vi "35Cl + 37Cl inj - 35Cl HE.vi"(6 "measure transmission?":bool, 7 "na/V 2":dbl=5000.0, 8 "error in":errorcluster, 9 "measure ss":bool=TRUE, 10 "field change wait(s)":u32=8, 11 "na/V":dbl=1000.0) -> (0 "error out":errorcluster, 1 "stable current 2":dbl format="%.2f", 3 "stable current":dbl=0.03723971270335772 format="%.2f", 4 "inj current":dbl format="%#_6e", 5 "INJ ss ratio":dbl=389.85458034298625 format="%#_6e")   [LabVIEW 2016]
uses:
  stable controls/stable cluster.ctl
  kubley/data acquisition 2009/beamline/controls/stable state combo.ctl
panel:
  in  "Start.Delay":dbl=2.0 format="%#_13g"
  in  "Charge State":dbl=3.0
  out "stable 1":dbl[](graph)=[-0.0009545581890180112, 0.0016222985467501813, 0.00033387017901426776, -0.0006324510969819727, -0.0009545581890180112, -0.002887200741629495, -0.0019208794652387398, 0.0006559772709758986, 0.00033387017901426776, -0.0009545581890180112, -0.0009545581890180112, -0.003853522018191701, -0.0012766652810727833, 0.002588619822359656, 0.0016222985467501813, 0.003554941097805747, 1.1763087034114085e-05, 0.0006559772709758986, 1.1763087034114085e-05, 0.00033387017901426776, -0.0012766652810727833, -0.0022429865573500296, 0.0029107269141931034, 0.0016222985467501813, -0.0032093078337977767, 0.0016222985467501813, -0.003531414925985161, 0.0006559772709758986, 0.0006559772709758986, -0.0022429865573500296, -0.00031034400496461514, 0.0009780843629190593, -0.00031034400496461514, 0.00033387017901426776, 0.00033387017901426776, -0.0012766652810727833, 0.0038770481895850487, 0.00033387017901426776, 0.001944405638638248, -0.0032093078337977767, -0.00031034400496461514, -0.0009545581890180112, -0.0009545581890180112, 0.001944405638638248, 1.1763087034114085e-05, 0.00033387017901426776, -0.0009545581890180112, 0.0013001914548438026, -0.0009545581890180112, 0.00033387017901426776, 0.0009780843629190593, -0.00031034400496461514, 0.001944405638638248, 0.0016222985467501813, -0.0012766652810727833, 0.00033387017901426776, -0.001598772373146342, 0.0013001914548438026, 0.0006559772709758986, 0.001944405638638248, -0.0019208794652387398, -0.0012766652810727833, -0.0006324510969819727, -0.0032093078337977767, 0.00033387017901426776, 0.0013001914548438026, 1.1763087034114085e-05, 0.002588619822359656, -0.0022429865573500296, -0.0006324510969819727, 0.0009780843629190593, 0.0009780843629190593, 0.003232834006008449, -0.001598772373146342, -0.0009545581890180112, -0.0009545581890180112, 0.0009780843629190593, 0.0029107269141931034, 0.0041991552813464075, 0.001944405638638248, 0.002266512730508055, 0.002588619822359656, -0.00031034400496461514, -0.0032093078337977767, -0.001598772373146342, 1.1763087034114085e-05, -0.002887200741629495, 1.1763087034114085e-05, -0.0019208794652387398, -0.00031034400496461514, -0.0009545581890180112, -0.0012766652810727833, 0.00033387017901426776, -0.0009545581890180112, -0.001598772373146342, 0.00033387017901426776, -0.0012766652810727833, -0.0006324510969819727, -0.001598772373146342, 0.0013001914548438026, -0.002565093649480264, 0.001944405638638248, -0.002565093649480264, -0.0009545581890180112, -0.001598772373146342, -0.001598772373146342, -0.001598772373146342, -0.0009545581890180112, 0.002588619822359656, -0.0019208794652387398, 1.1763087034114085e-05, 0.002266512730508055, 0.0041991552813464075, 0.00033387017901426776, 0.002588619822359656, -0.0032093078337977767, -0.0022429865573500296, 0.00033387017901426776, -0.0022429865573500296, -0.0012766652810727833, 1.1763087034114085e-05, -0.0006324510969819727, 0.0006559772709758986, -0.00031034400496461514, 1.1763087034114085e-05, -0.0006324510969819727, -0.0009545581890180112, 0.0013001914548438026, -0.0012766652810727833, -0.0012766652810727833, 0.002266512730508055, -0.0012766652810727833, -0.0012766652810727833, 0.0009780843629190593, -0.0019208794652387398, -0.001598772373146342, -0.002565093649480264, -0.0012766652810727833, -0.0012766652810727833, -0.0032093078337977767, -0.0022429865573500296, 0.0009780843629190593, -0.0006324510969819727, 1.1763087034114085e-05, -0.00031034400496461514, 0.00033387017901426776, 0.0013001914548438026, -0.0006324510969819727, -0.002565093649480264, -0.0006324510969819727, -0.00031034400496461514, -0.0019208794652387398, 0.002588619822359656, -0.003531414925985161, -0.00031034400496461514, -0.0006324510969819727, 0.0009780843629190593, 1.1763087034114085e-05, -0.0009545581890180112, 0.00033387017901426776, 0.0009780843629190593, 0.001944405638638248, 0.00033387017901426776, -0.00031034400496461514, 0.0016222985467501813, 0.0009780843629190593, -0.0006324510969819727, -0.0012766652810727833, 0.00033387017901426776, -0.0019208794652387398, -0.001598772373146342, -0.0006324510969819727, 0.0013001914548438026, -0.0032093078337977767, -0.00031034400496461514, -0.003531414925985161, 0.00033387017901426776, -0.002565093649480264, -0.0012766652810727833, -0.0006324510969819727, 0.0029107269141931034, 0.0006559772709758986, -0.0009545581890180112, 0.0013001914548438026, -0.00031034400496461514, -0.002887200741629495, 0.003232834006008449, -0.0012766652810727833, 0.0016222985467501813, 0.002588619822359656, 0.00033387017901426776, 0.003232834006008449]
  in  "stable data in":T1={"injector current"=1.0, "offset current"=1.0, "ss inj ratio"=1.0, "ss offset ratio"=1.0, "transmission"=1.0, "2nd offset current"=1.0}
  out "stable data out":T1={"injector current"=1.0, "offset current"=0.03723971270335772, "ss inj ratio"=389.85458034298625, "ss offset ratio"=inf, "transmission"=0.5319958957622531, "2nd offset current"=1.0}
  out "stable 2":dbl[](graph)
  in  "inj current 4":dbl=1.8438580000000002e-12
  out "inj current 3":dbl=0.002565059 format="%#_6e"
  in  "inj current 2":dbl=1.8438580000000002e-12
  out "step":string="run"
  in  "measure stable":bool
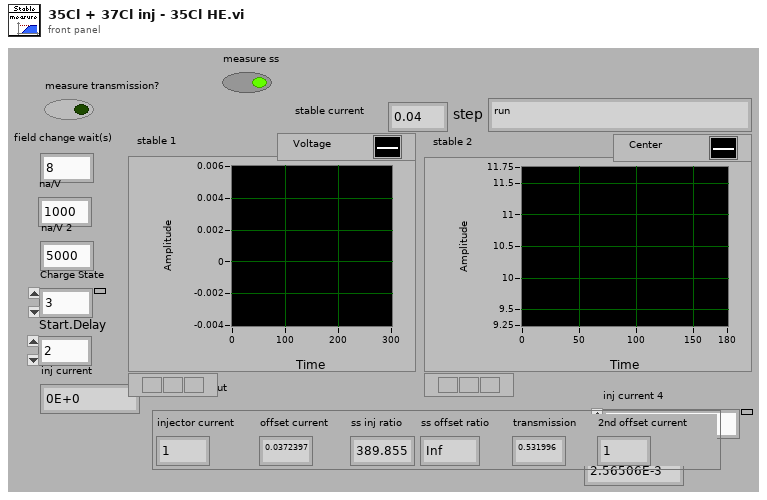
[diagram p1: front panel]
types:
  T1 = typedef "stable cluster.ctl" = cluster{"injector current":dbl, "offset current":dbl, "ss inj ratio":dbl, "ss offset ratio":dbl, "transmission":dbl, "2nd offset current":dbl}
  T2 = typedef "stable state combo.ctl" = string
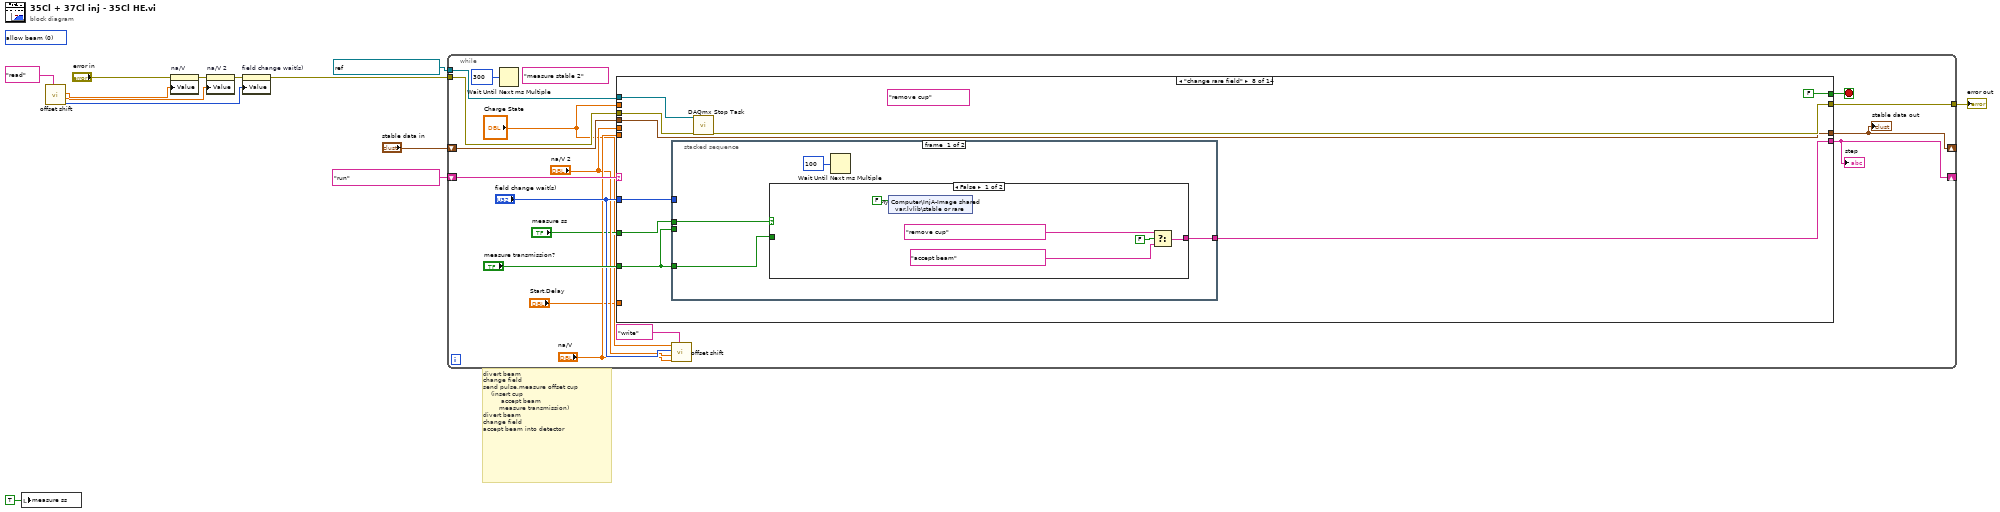
[diagram p0: block diagram]
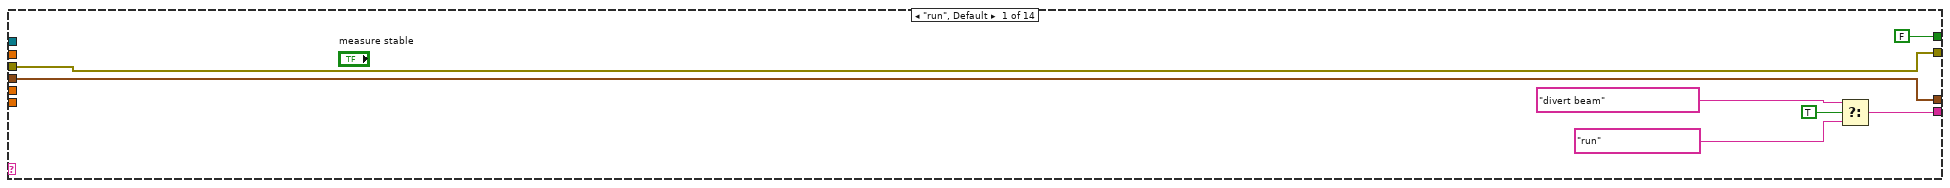
[diagram p2: hidden frame]
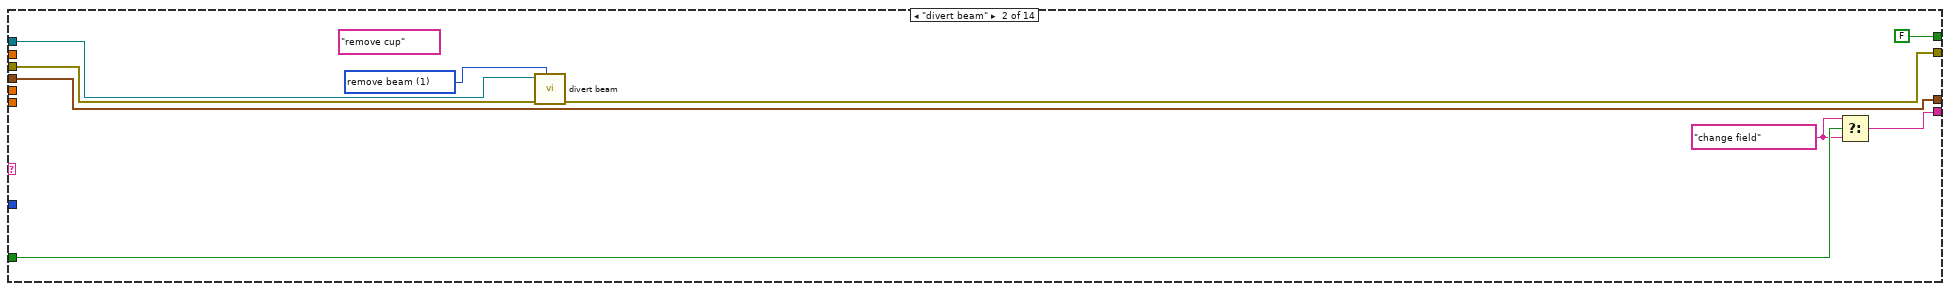
[diagram p3: hidden frame]
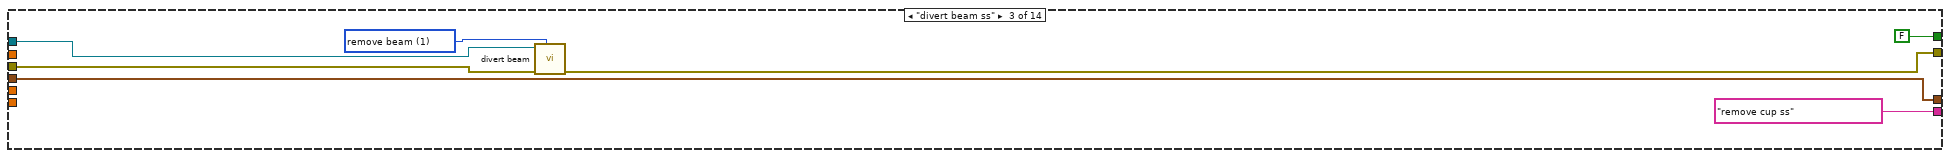
[diagram p4: hidden frame]
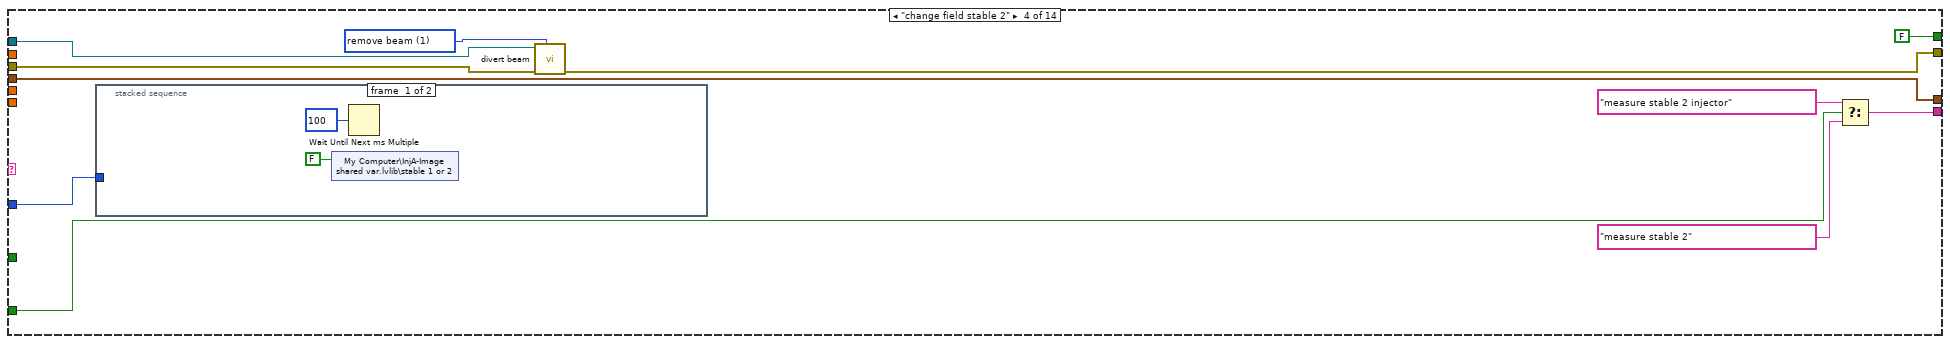
[diagram p5: hidden frame]
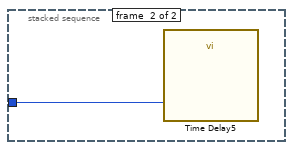
[diagram p6: hidden frame]
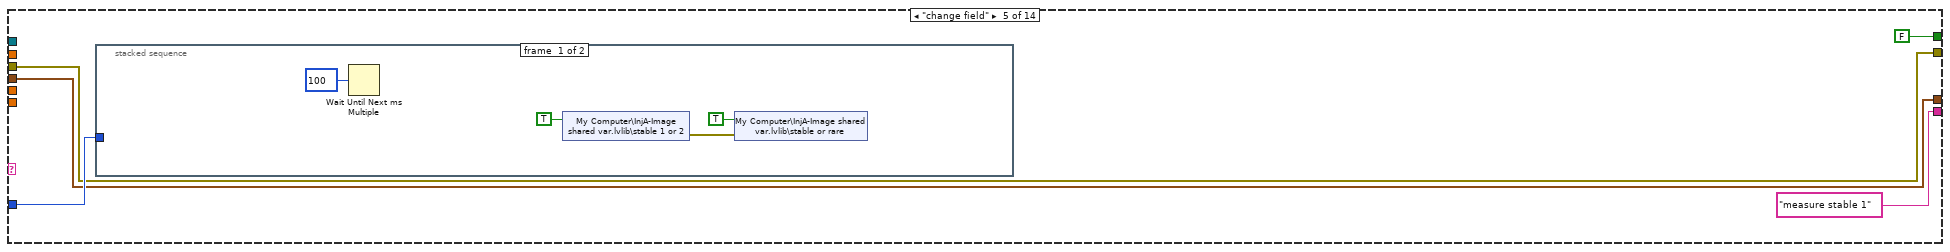
[diagram p7: hidden frame]
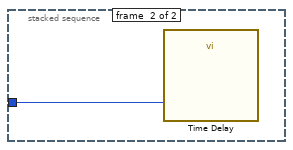
[diagram p8: hidden frame]
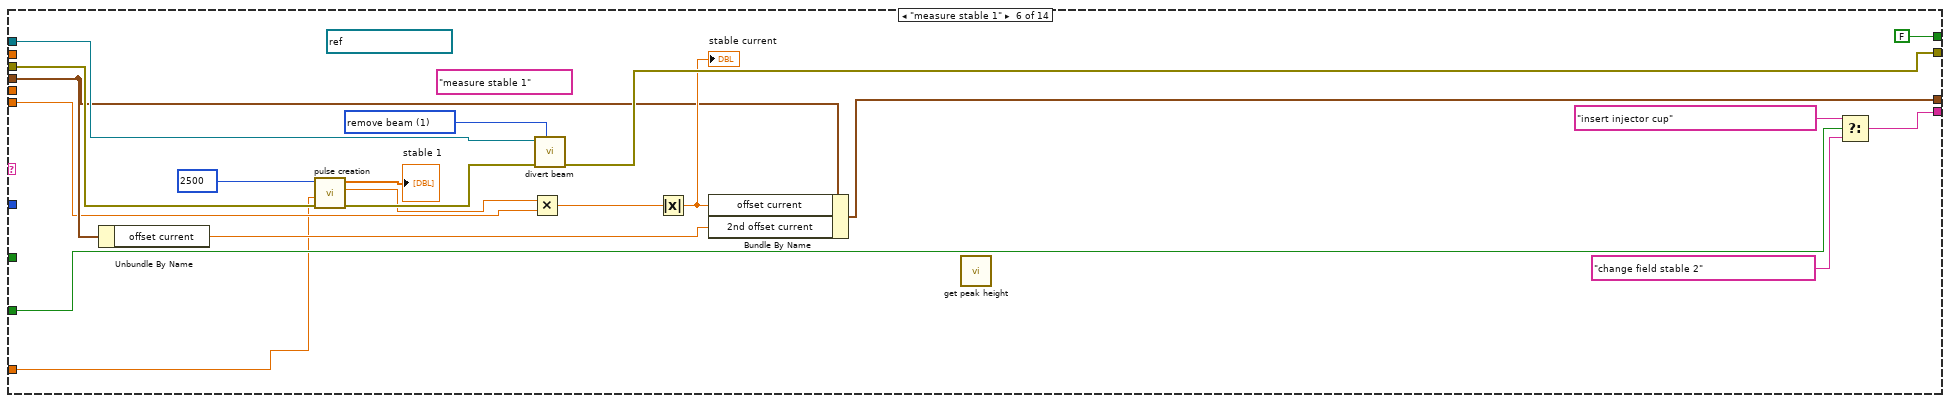
[diagram p9: hidden frame]
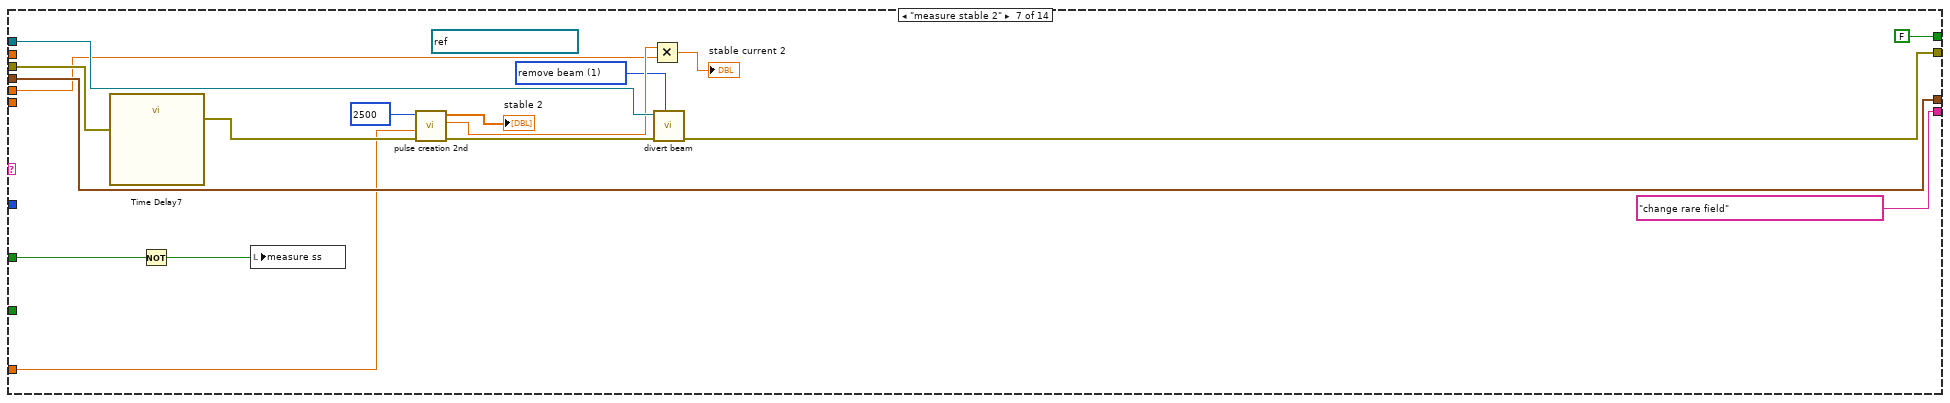
[diagram p10: hidden frame]
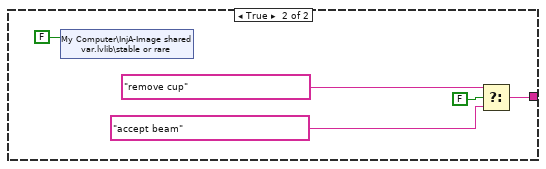
[diagram p11: hidden frame]
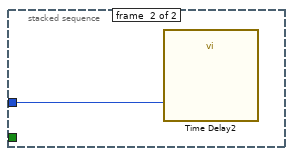
[diagram p12: hidden frame]
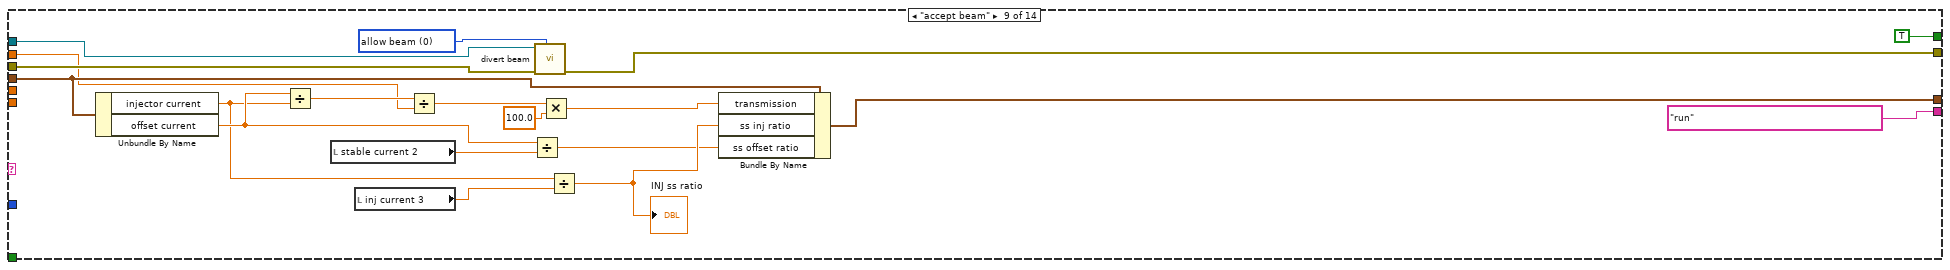
[diagram p13: hidden frame]
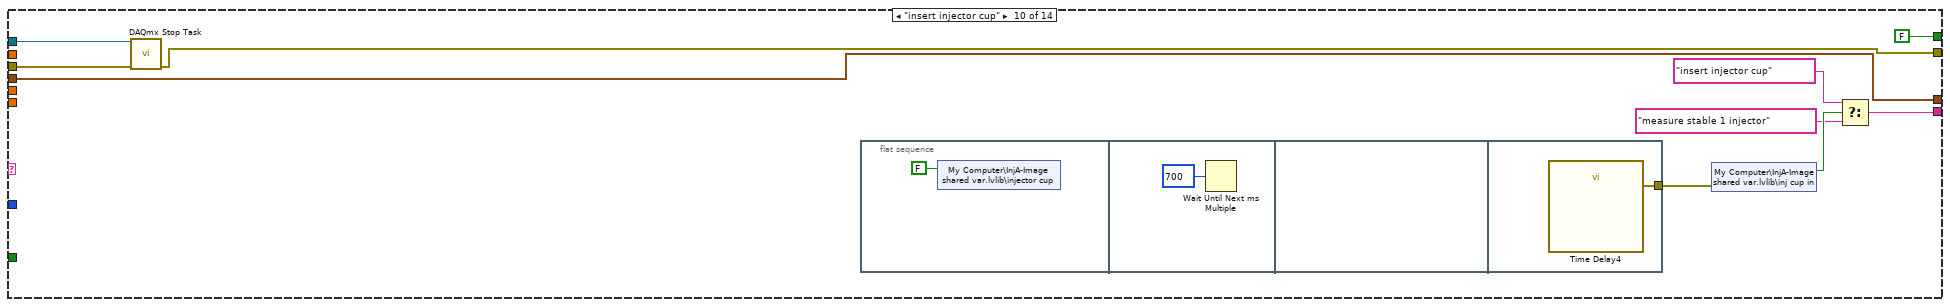
[diagram p14: hidden frame]
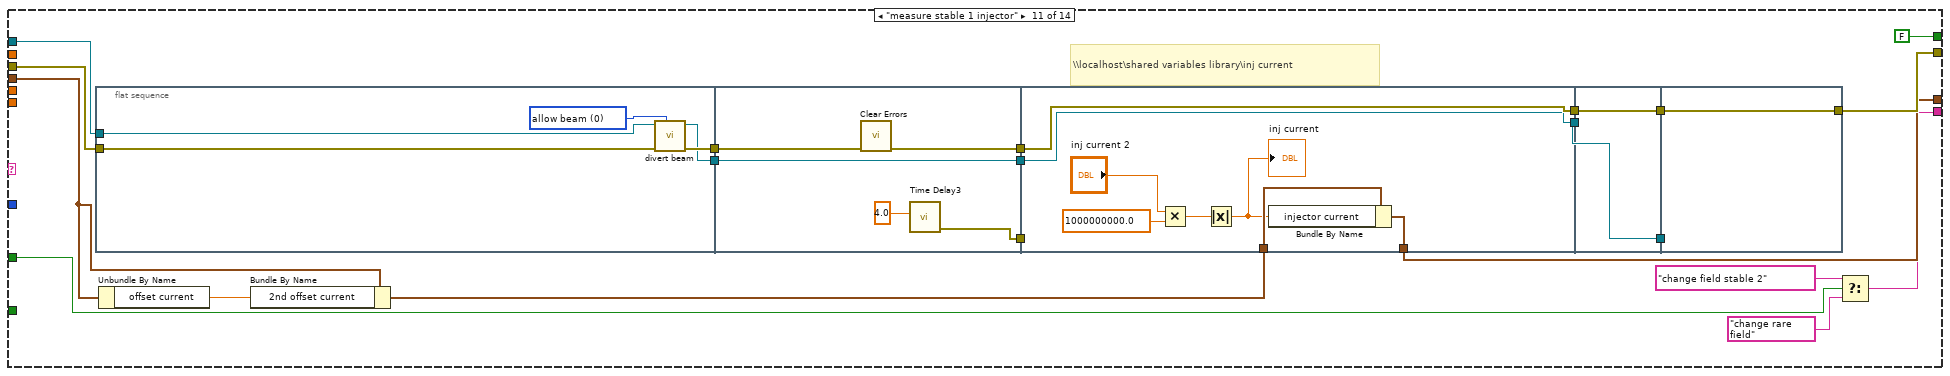
[diagram p15: hidden frame]
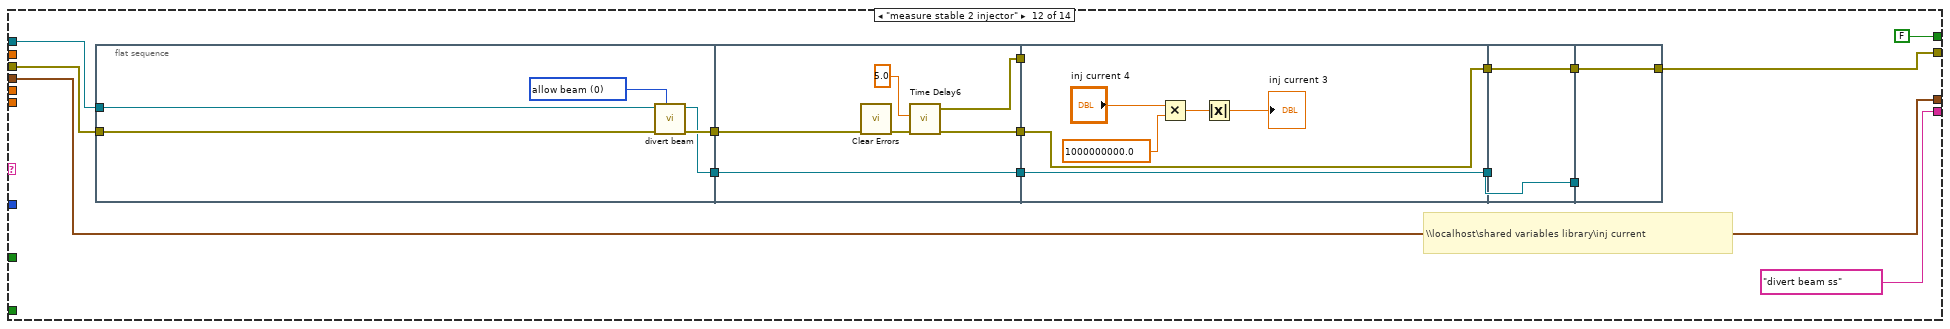
[diagram p16: hidden frame]
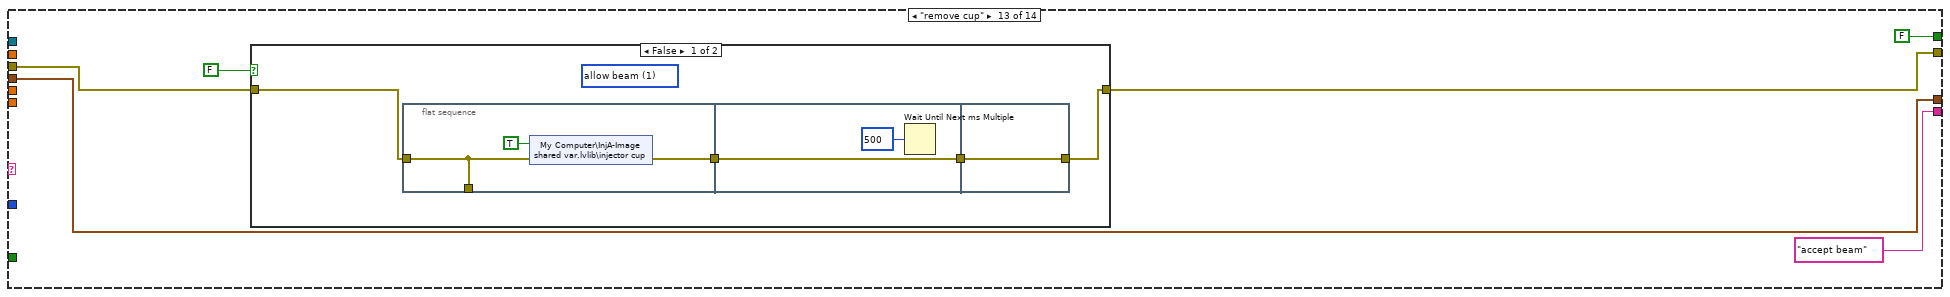
[diagram p17: hidden frame]
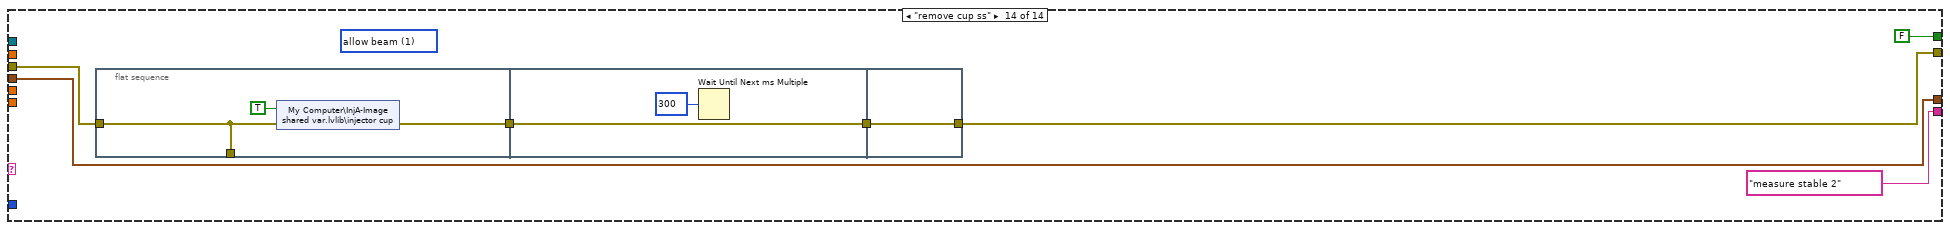
[diagram p19: hidden frame]
diagram:
  (unwired) u16 0 items=["allow beam", "remove beam"] ("divert beam? 2")
  # "divert beam\nchange field\nsend pulse,measure offset cup\n    (insert cup\n         accept beam\n        measure transmission)\ndivert beam\nchange field\naccept beam into detector"
  n1 = local write "measure ss"(TRUE ("measure ss")) -> ()
  n2 = call "offset shift.vi"("read writ"="read") -> ("field change wait(s) out"=w6:u32, "na/V 2out"=w7:dbl, "na/V out"=w8:dbl)  [unwired: 7 in, 1 out]
  n3 = property on="na/V" class="DigNum (strict)"(error in="error in", "Value"=w8) -> (error out=w5:errorcluster)  [unwired: 1 in, 1 out]
  n4 = property on="na/V 2" class="DigNum (strict)"(error in=w5, "Value"=w7) -> (error out=w4:errorcluster)  [unwired: 1 in, 1 out]
  n5 = property on="field change wait(s)" class="DigNum (strict)"(error in=w4, "Value"=w6) -> (error out=w3:errorcluster)  [unwired: 1 in, 1 out]
  n6 = while {
    shift-right: [w29] -> _
    shift-left: T2 "run" ("stable measurement type") -> [w30]
    tunnel: refnum<k21> "stable current output" ("task/channels in") -> [w28]
    tunnel: [w26] -> w11
    tunnel: w3 -> [w25]
    shift-right: [w21] -> _
    shift-left: "stable data in" -> [w22]
    stop <- w24 stop-if-true
    (unwired) T2 "measure stable 2" ("stable measurement type")
    n7 = Wait Until Next ms Multiple(millisecond multiple=u32 300) -> ()  [unwired: 1 out]
    n8 = case shown="\"change rare field\"" w30 {
      tunnel: [w35 w41 T2 "remove cup ss" ("stable measurement type") w55 T2 "measure stable 1" ("stable measurement type") w88 T2 "change rare field" ("stable measurement type") w116 T2 "run" ("stable measurement type") w161 w171 T2 "divert beam ss" ("stable measurement type") T2 "accept beam" ("stable measurement type") T2 "measure stable 2" ("stable measurement type")] -> w29
      tunnel: w28 -> [_ w46 w53 w64 _ w93 w111 w121 w157 w166 w188 w225 _ _]
      tunnel: "field change wait(s)" -> [_ _ _ w60 w71 _ _ w123 _ _ _ _ _ _]
      tunnel: [FALSE ("stop") FALSE ("stop") FALSE ("stop") FALSE ("stop") FALSE ("stop") FALSE ("stop") FALSE ("stop") FALSE ("stop") TRUE ("stop") FALSE ("stop") FALSE ("stop") FALSE ("stop") FALSE ("stop") FALSE ("stop")] -> w24
      tunnel: [w32 w44 w51 w62 w69 w90 w109 w119 w153 w164 w179 w216 w249 w267] -> w26
      tunnel: w25 -> [w32 w43 w50 w61 w69 w94 w105 w120 w154 w165 w185 w222 w250 w268]
      tunnel: "measure transmission?" -> [_ _ _ w57 _ w92 _ w117 _ _ _ _ _ _]
      tunnel: "measure ss" -> [_ w42 _ _ _ _ w107 w118 _ _ w178 _ _ _]
      tunnel: w22 -> [w31 w38 w47 w58 w68 w82 w100 w115 w149 w160 w175 w214 w247 w264]
      tunnel: [w31 w38 w47 w58 w68 w83 w100 w115 w148 w160 w177 w214 w247 w264] -> w21
      tunnel: "Charge State" -> [_ _ _ _ _ _ _ _ w144 _ _ _ _ _]
      tunnel: "na/V" -> [_ _ _ _ _ w80 _ _ _ _ _ _ _ _]
      tunnel: "na/V 2" -> [_ _ _ _ _ _ w99 _ _ _ _ _ _ _]
      tunnel: "Start.Delay" -> [_ _ _ _ _ w78 w98 _ _ _ _ _ _ _]
      frame "run", Default {
        n9 = Select(t=T2 "divert beam" ("stable measurement type"), s=TRUE, f=T2 "run" ("stable measurement type")) -> (s? t:f=w35:T2)
      }
      frame "divert beam" {
        w39 = u16 1 items=["allow beam", "remove beam"] ("divert beam? 2")
        (unwired) T2 "remove cup" ("stable measurement type")
        w40 = T2 "change field" ("stable measurement type")
        n10 = call "divert beam.vi"("divert beam?"=w39, "error in"=w43, "task/channels in"=w46) -> ("error out"=w44:errorcluster)  [unwired: 7 in, 1 out]
        n11 = Select(t=w40, s=w42, f=w40) -> (s? t:f=w41:T2)
      }
      frame "divert beam ss" {
        w48 = u16 1 items=["allow beam", "remove beam"] ("divert beam? 2")
        n12 = call "divert beam.vi"("divert beam?"=w48, "error in"=w50, "task/channels in"=w53) -> ("error out"=w51:errorcluster)  [unwired: 7 in, 1 out]
      }
      frame "change field stable 2" {
        w59 = u16 1 items=["allow beam", "remove beam"] ("divert beam? 2")
        n13 = stacked-sequence {
          tunnel: w60 -> [_ w67]
          frame #0 {
            n14 = shared-variable "My Computer\\InjA-Image shared var.lvlib\\stable 1 or 2"(FALSE ("stable or rare")) -> ()  [unwired: 1 in, 1 out]
            n15 = Wait Until Next ms Multiple(millisecond multiple=u32 100) -> ()  [unwired: 1 out]
          }
          frame #1 {
            n16 = call "Time Delay5"("Delay Time (s)"=w67) -> ()  [unwired: 10 in, 1 out]
          }
        }
        n17 = call "divert beam.vi"("divert beam?"=w59, "error in"=w61, "task/channels in"=w64) -> ("error out"=w62:errorcluster)  [unwired: 7 in, 1 out]
        n18 = Select(t=T2 "measure stable 2 injector" ("stable measurement type"), s=w57, f=T2 "measure stable 2" ("stable measurement type")) -> (s? t:f=w55:T2)
      }
      frame "change field" {
        n19 = stacked-sequence {
          tunnel: w71 -> [_ w77]
          frame #0 {
            n20 = Wait Until Next ms Multiple(millisecond multiple=u32 100) -> ()  [unwired: 1 out]
            n21 = shared-variable "My Computer\\InjA-Image shared var.lvlib\\stable 1 or 2"(TRUE ("stable or rare")) -> (error out=w73:errorcluster)  [unwired: 1 in]
            n22 = shared-variable "My Computer\\InjA-Image shared var.lvlib\\stable or rare"(TRUE ("stable or rare"), error in=w73) -> ()  [unwired: 1 out]
          }
          frame #1 {
            n23 = call "Time Delay"("Delay Time (s)"=w77) -> ()  [unwired: 10 in, 1 out]
          }
        }
      }
      frame "measure stable 1" {
        w85 = u16 1 items=["allow beam", "remove beam"] ("divert beam? 2")
        (unwired) refnum<k21> "stable currents" ("task/channels in")
        (unwired) T2 "measure stable 1" ("stable measurement type")
        n24 = Unbundle By Name(w82) -> ("offset current"=w81:dbl)
        n25 = call "pulse creation.vi"("error in"=w94, "Start.Delay"=w78, "chopper width(usec)"=u32 2500) -> ("error out"=w96:errorcluster, "mean"=w86:dbl, "Waveform Graph 2"=→"stable 1":dbl[])  [unwired: 4 in, 2 out]
        n26 = Multiply(x=w86, y=w80) -> (x*y=w87:dbl)
        n27 = call "divert beam.vi"("divert beam?"=w85, "error in"=w96, "task/channels in"=w93) -> ("error out"=w90:errorcluster)  [unwired: 7 in, 1 out]
        n28 = Absolute Value(x=w87) -> (abs(x)=w84:dbl)
        "stable current" <- w84
        n29 = Bundle By Name(cluster=w82, "offset current"=w84, "2nd offset current"=w81) -> (w83:T1)
        n30 = call "get peak height.vi"() -> ()  [unwired: 8 in, 4 out]
        n31 = Select(t=T2 "insert injector cup" ("stable measurement type"), s=w92, f=T2 "change field stable 2" ("stable measurement type")) -> (s? t:f=w88:T2)
      }
      frame "measure stable 2" {
        w101 = u16 1 items=["allow beam", "remove beam"] ("divert beam? 2")
        (unwired) refnum<k21> "secondary current" ("task/channels in")
        n32 = call "Time Delay7"("error in (no error)"=w105) -> ("error out"=w104:errorcluster)  [unwired: 10 in]
        n33 = Not(x=w107) -> (.not. x?=w106:bool)
        n34 = local write "measure ss"(w106) -> ()
        n35 = call "pulse creation 2nd.vi"("error in"=w104, "Start.Delay"=w98, "chopper width(usec)"=u32 2500) -> ("error out"=w113:errorcluster, "mean"=w102:dbl, "Waveform Graph"=→"stable 2":dbl[])  [unwired: 6 in]
        n36 = Multiply(x=w102, y=w99) -> (x*y=→"stable current 2":dbl)
        n37 = call "divert beam.vi"("divert beam?"=w101, "error in"=w113, "task/channels in"=w111) -> ("error out"=w109:errorcluster)  [unwired: 7 in, 1 out]
      }
      frame "change rare field" {
        (unwired) T2 "remove cup" ("stable measurement type")
        n38 = stacked-sequence {
          tunnel: w123 -> [_ w138]
          tunnel: w118 -> [w126 _]
          tunnel: w117 -> [w125 _]
          tunnel: w117 -> [_ _]
          tunnel: [w124 _] -> w116
          frame #0 {
            n39 = case shown="False" w126 {
              tunnel: w125 -> [_ _]
              tunnel: [w129 w134] -> w124
              frame False {
                n40 = shared-variable "My Computer\\InjA-Image shared var.lvlib\\stable or rare"(FALSE ("stable or rare")) -> ()  [unwired: 1 in, 1 out]
                n41 = Select(t=T2 "remove cup" ("stable measurement type"), s=FALSE ("stable or rare"), f=T2 "accept beam" ("stable measurement type")) -> (s? t:f=w129:T2)
              }
              frame True {
                n42 = shared-variable "My Computer\\InjA-Image shared var.lvlib\\stable or rare"(FALSE ("stable or rare")) -> ()  [unwired: 1 in, 1 out]
                n43 = Select(t=T2 "remove cup" ("stable measurement type"), s=FALSE ("stable or rare"), f=T2 "accept beam" ("stable measurement type")) -> (s? t:f=w134:T2)
              }
            }
            n44 = Wait Until Next ms Multiple(millisecond multiple=u32 100) -> ()  [unwired: 1 out]
          }
          frame #1 {
            n45 = call "Time Delay2"("Delay Time (s)"=w138) -> ()  [unwired: 10 in, 1 out]
          }
        }
        n46 = call <vilib>:"DAQmx Stop Task.vi"("task/channels in"=w121, "error in"=w120) -> ("error out"=w119:errorcluster)  [unwired: 12 in, 1 out]
      }
      frame "accept beam" {
        w151 = u16 0 items=["allow beam", "remove beam"] ("divert beam? 2")
        n47 = Unbundle By Name(w149) -> ("injector current"=w140:dbl, "offset current"=w141:dbl)
        n48 = Divide(x=w141, y=w140) -> (x/y=w150:dbl)
        n49 = local read "stable current 2"() -> (w142:dbl)
        n50 = local read "inj current 3"() -> (w152:dbl)
        n51 = Divide(x=w150, y=w144) -> (x/y=w147:dbl)
        n52 = Divide(x=w141, y=w142) -> (x/y=w139:dbl)
        n53 = call "divert beam.vi"("divert beam?"=w151, "error in"=w154, "task/channels in"=w157) -> ("error out"=w153:errorcluster)  [unwired: 7 in, 1 out]
        n54 = Multiply(x=w147, y=100.0) -> (x*y=w145:dbl)
        n55 = Divide(x=w140, y=w152) -> (x/y=w143:dbl)
        "INJ ss ratio" <- w143
        n56 = Bundle By Name(cluster=w149, "transmission"=w145, "ss inj ratio"=w143, "ss offset ratio"=w139) -> (w148:T1)
      }
      frame "insert injector cup" {
        n57 = call <vilib>:"DAQmx Stop Task.vi"("task/channels in"=w166, "error in"=w165) -> ("error out"=w164:errorcluster)  [unwired: 12 in, 1 out]
        n58 = flat-sequence {
          tunnel: [w170] -> w163
          frame #0 {
            n59 = shared-variable "My Computer\\InjA-Image shared var.lvlib\\injector cup"(FALSE ("injector cup")) -> ()  [unwired: 1 in, 1 out]
          }
          frame #1 {
            n60 = Wait Until Next ms Multiple(millisecond multiple=u32 700) -> ()  [unwired: 1 out]
          }
          frame #2 {
          }
          frame #3 {
            n61 = call "Time Delay4"() -> ("error out"=w170:errorcluster)  [unwired: 11 in]
          }
        }
        n62 = shared-variable "My Computer\\InjA-Image shared var.lvlib\\inj cup in"(error in=w163) -> (w162:bool)  [unwired: 1 out]
        n63 = Select(t=T2 "insert injector cup" ("f"), s=w162, f=T2 "measure stable 1 injector" ("stable measurement type")) -> (s? t:f=w161:T2)
      }
      frame "measure stable 1 injector" {
        # "\\\\localhost\\shared variables library\\inj current"
        n64 = flat-sequence {
          tunnel: w188 -> [w196]
          tunnel: [w195] -> w189
          tunnel: [w193] -> w186
          tunnel: w185 -> [w194]
          tunnel: [w199] -> w190
          tunnel: w189 -> [w200]
          tunnel: [w201] -> w187
          tunnel: w186 -> [w201]
          tunnel: [w197] -> w180
          tunnel: [w209] -> w184
          tunnel: w190 -> [w209]
          tunnel: [w208] -> w182
          tunnel: w187 -> [w208]
          tunnel: w180 -> [_]
          tunnel: w174 -> [w207]
          tunnel: [w206] -> w177
          tunnel: w184 -> [w211]
          tunnel: [w211] -> w183
          tunnel: w182 -> [w210]
          tunnel: [w210] -> w181
          tunnel: w183 -> [w212]
          tunnel: w181 -> [_]
          tunnel: [w212] -> w179
          frame #0 {
            w192 = u16 0 items=["allow beam", "remove beam"] ("divert beam? 2")
            n65 = call "divert beam.vi"("divert beam?"=w192, "error in"=w194, "task/channels in"=w196) -> ("error out"=w195:errorcluster, "task out"=w193:refnum<k21>)  [unwired: 7 in]
          }
          frame #1 {
            n66 = call <vilib>:"Clear Errors.vi"("error in (no error)"=w200) -> ("error out"=w199:errorcluster)  [unwired: 5 in, 1 out]
            n67 = call "Time Delay3"("Delay Time (s)"=4.0) -> ("error out"=w197:errorcluster)  [unwired: 10 in]
          }
          frame #2 {
            n68 = Multiply(x="inj current 2", y=1000000000.0) -> (x*y=w203:dbl)
            n69 = Absolute Value(x=w203) -> (abs(x)=w202:dbl)
            "inj current" <- w202
            n70 = Bundle By Name(cluster=w207, "injector current"=w202) -> (w206:T1)
          }
          frame #3 {
          }
          frame #4 {
          }
        }
        n71 = Unbundle By Name(w175) -> ("offset current"=w176:dbl)
        n72 = Bundle By Name(cluster=w175, "2nd offset current"=w176) -> (w174:T1)
        n73 = Select(t=T2 "change field stable 2" ("stable measurement type"), s=w178, f=T2 "change rare field" ("stable measurement type")) -> (s? t:f=w171:T2)
      }
      frame "measure stable 2 injector" {
        # "\\\\localhost\\shared variables library\\inj current"
        n74 = flat-sequence {
          tunnel: w225 -> [w232]
          tunnel: [w231] -> w226
          tunnel: [w229] -> w223
          tunnel: w222 -> [w230]
          tunnel: w226 -> [w236]
          tunnel: [w237] -> w224
          tunnel: w223 -> [w237]
          tunnel: [w233] -> w217
          tunnel: [w233] -> w213
          tunnel: [w243] -> w221
          tunnel: [w242] -> w219
          tunnel: w224 -> [w242]
          tunnel: w217 -> [_]
          tunnel: w213 -> [w243]
          tunnel: w221 -> [w245]
          tunnel: [w245] -> w220
          tunnel: w219 -> [w244]
          tunnel: [w244] -> w218
          tunnel: w220 -> [w246]
          tunnel: w218 -> [_]
          tunnel: [w246] -> w216
          frame #0 {
            w228 = u16 0 items=["allow beam", "remove beam"] ("divert beam? 2")
            n75 = call "divert beam.vi"("divert beam?"=w228, "error in"=w230, "task/channels in"=w232) -> ("error out"=w231:errorcluster, "task out"=w229:refnum<k21>)  [unwired: 7 in]
          }
          frame #1 {
            n76 = call <vilib>:"Clear Errors.vi"("error in (no error)"=w236) -> ("error out"=w234:errorcluster)  [unwired: 5 in, 1 out]
            n77 = call "Time Delay6"("error in (no error)"=w234, "Delay Time (s)"=5.0) -> ("error out"=w233:errorcluster)  [unwired: 9 in]
          }
          frame #2 {
            n78 = Multiply(x="inj current 4", y=1000000000.0) -> (x*y=w240:dbl)
            n79 = Absolute Value(x=w240) -> (abs(x)=→"inj current 3":dbl)
          }
          frame #3 {
          }
          frame #4 {
          }
        }
      }
      frame "remove cup" {
        n80 = case shown="False" FALSE {
          tunnel: w250 -> [w254 w263]
          tunnel: [w253 w263] -> w249
          frame False {
            (unwired) u16 1 items=["divert beam", "allow beam"] ("divert beam? 2")
            n81 = flat-sequence {
              tunnel: [w257] -> _
              tunnel: w254 -> [w257]
              tunnel: [w258] -> w256
              tunnel: [w260] -> w255
              tunnel: w256 -> [w260]
              tunnel: w255 -> [w262]
              tunnel: [w262] -> w253
              frame #0 {
                n82 = shared-variable "My Computer\\InjA-Image shared var.lvlib\\injector cup"(TRUE ("injector cup"), error in=w257) -> (error out=w258:errorcluster)
              }
              frame #1 {
                n83 = Wait Until Next ms Multiple(millisecond multiple=u32 500) -> ()  [unwired: 1 out]
              }
              frame #2 {
              }
            }
          }
          frame True {
          }
        }
      }
      frame "remove cup ss" {
        (unwired) u16 1 items=["divert beam", "allow beam"] ("divert beam? 2")
        n84 = flat-sequence {
          tunnel: [w271] -> _
          tunnel: w268 -> [w271]
          tunnel: [w272] -> w266
          tunnel: [w274] -> w265
          tunnel: w266 -> [w274]
          tunnel: w265 -> [w276]
          tunnel: [w276] -> w267
          frame #0 {
            n85 = shared-variable "My Computer\\InjA-Image shared var.lvlib\\injector cup"(TRUE ("injector cup"), error in=w271) -> (error out=w272:errorcluster)
          }
          frame #1 {
            n86 = Wait Until Next ms Multiple(millisecond multiple=u32 300) -> ()  [unwired: 1 out]
          }
          frame #2 {
          }
        }
      }
    }
    "step" <- w29
    "stable data out" <- w21
    n87 = call "offset shift.vi"("read writ"="write", "na/V"="na/V", "na/V 2"="na/V 2", "field change wait(s)"="field change wait(s)", "charge state"="Charge State") -> ()  [unwired: 3 in, 4 out]
  }
  "error out" <- w11
